vi "FollowAttackerRole.vi"(8 "error in (no error)":errorcluster, 10 "Game in":refnum<class "Game.lvclass">, 11 "FollowAttackerRole in":refnum<class "FollowAttackerRole.lvclass">) -> (0 "error out":errorcluster, 1 "Game out":refnum<class "Game.lvclass">, 2 "Robot out":refnum<class "Robot.lvclass">, 3 "FollowAttackerRole out":refnum<class "FollowAttackerRole.lvclass">)   [LabVIEW 2018, in "FollowAttackerRole.lvclass"]
uses:
  FollowAttackerRole.lvclass
  C:/Users/nicolas.oliveira/roboime/SSL_AI/Role_class/Role.lvclass
  Game_class/Game.lvclass
  Robot_class/Robot.lvclass
  Role_class/Role.lvclass/Role.ctl
  TestTactic_class/States.ctl
  Tacticbook_class/Tacticbook.lvclass/Tacticbook.ctl
  FollowAttackerTactic_class/FollowAttackerTactic.lvclass/FollowAttackerTactic.ctl
  Tacticbook_class/Read FollowAttackerTactic.vi
  FollowAttackerTactic_class/Read States.vi
  Tacticbook_class/Write FollowAttackerTactic.vi
  Role_class/Read Tacticbook.vi
  Role_class/Write Tacticbook.vi
  Role_class/Write tactic_index.vi
  Role_class/Read RobotRef.vi
  Tacticbook_class/Tacticbook.lvclass
  FollowAttackerTactic_class/FollowAttackerTactic.lvclass
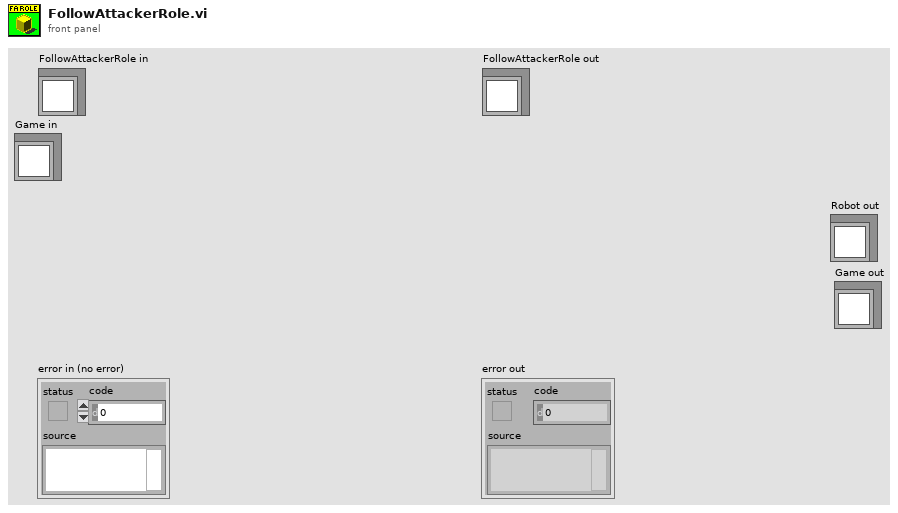
[diagram p1: front panel]
types:
  T1 = typedef "States.ctl" = enum16{"State 1", "Exit"}
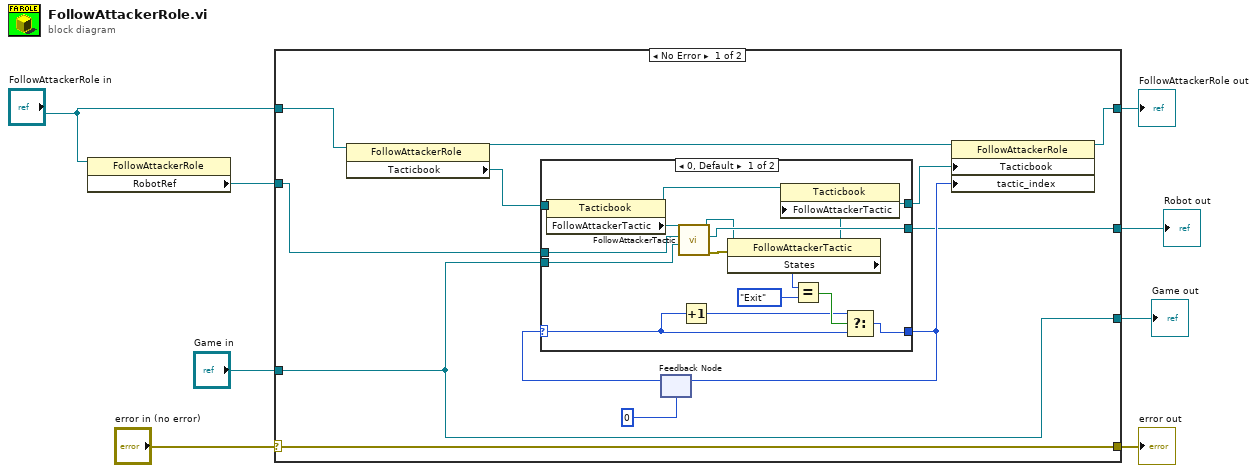
[diagram p0: block diagram]
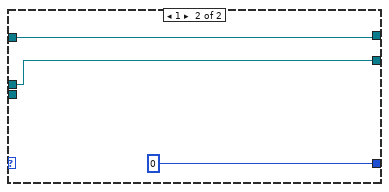
[diagram p2: hidden frame]
diagram:
  n1 = property class="FollowAttackerRole"(reference="FollowAttackerRole in") -> ("RobotRef"=w4:refnum<class "Robot.lvclass">)  [unwired: 1 in, 2 out]
  n2 = case shown="No Error" "error in (no error)" {
    selector: "error in (no error)" -> [w20 w43]
    tunnel: [w20 w43] -> w7
    tunnel: [w12 w42] -> w6
    tunnel: "FollowAttackerRole in" -> [w13 w42]
    tunnel: w4 -> [w9 w41]
    tunnel: [w11 w41] -> w3
    tunnel: [w10 w40] -> w2
    tunnel: "Game in" -> [w10 w40]
    frame No Error {
      n3 = property class="FollowAttackerRole"(reference=w13) -> (reference out=w19:refnum<class "FollowAttackerRole.lvclass">, "Tacticbook"=w16:refnum<class "Tacticbook.lvclass">)  [unwired: 1 in, 1 out]
      n4 = feedback #1(0) -> (w17:i32)
      n5 = case shown="0, Default" w17 {
        selector: w17 -> [w26 _]
        tunnel: [w27 0] -> w15
        tunnel: w16 -> [w36 w37]
        tunnel: w9 -> [w34 w39]
        tunnel: [w33 w39] -> w11
        tunnel: [w22 w37] -> w14
        tunnel: w10 -> [w21 _]
        frame 0, Default {
          n6 = property class="Tacticbook"(reference=w36) -> (reference out=w24:refnum<class "Tacticbook.lvclass">, "FollowAttackerTactic"=w35:refnum<class "FollowAttackerTactic.lvclass">)  [unwired: 1 in, 1 out]
          n7 = call-dynamic "FollowAttackerTactic.vi"("Game in"=w21, "Robot"=w34, "FollowAttackerTactic in"=w35) -> ("error out"=w32:errorcluster, "Robot out"=w33:refnum<class "Robot.lvclass">, "FollowAttackerTactic out"=w31:refnum<class "FollowAttackerTactic.lvclass">)  [unwired: 6 in]
          n8 = Increment(x=w26) -> (x+1=w25:i32)
          n9 = property class="FollowAttackerTactic"(reference=w31, error in=w32) -> (reference out=w23:refnum<class "FollowAttackerTactic.lvclass">, "States"=w30:enum16{"Exit", "FollowAttacker"})  [unwired: 1 out]
          n10 = property class="Tacticbook"(reference=w24, "FollowAttackerTactic"=w23) -> (reference out=w22:refnum<class "Tacticbook.lvclass">)  [unwired: 1 in, 1 out]
          n11 = Equal?(x=w30, y=States."Exit") -> (x = y?=w28:bool)
          n12 = Select(t=w25, s=w28, f=w26) -> (s? t:f=w27:i32)
        }
        frame 1 {
        }
      }
      n13 = feedback-in #1(w15) -> ()
      n14 = property class="FollowAttackerRole"(reference=w19, "Tacticbook"=w14, "tactic_index"=w15) -> (reference out=w12:refnum<class "FollowAttackerRole.lvclass">)  [unwired: 1 in, 1 out]
    }
    frame Error {
    }
  }
  "error out" <- w7
  "FollowAttackerRole out" <- w6
  "Robot out" <- w3
  "Game out" <- w2
